vi "Simulated Car Client.vi"(7 "stop signal":refnum<user-event>, 10 "project namespace":string="LabVIEWDemo", 11 "Client Name":string="Car") -> ()   [LabVIEW 2017]
uses:
  Car/Car State -- enum.ctl
  <vilib>/LabVIEW Open Source Project/MQTT Broker/Client/Client.lvclass
  C:/Program Files (x86)/National Instruments/LabVIEW 2017/vi.lib/LabVIEW Open Source Project/MQTT Broker/MQTT_Base/MQTT_Base.lvclass
  <vilib>/LabVIEW Open Source Project/MQTT Broker/Control Packets/PUBLISH/PUBLISH.lvclass
  C:/Program Files (x86)/National Instruments/LabVIEW 2017/vi.lib/LabVIEW Open Source Project/MQTT Broker/Control Packets/ControlPacket/ControlPacket.lvclass
  Node Type -- enum.ctl
  TrafficMap/TrafficMap.lvclass
  RequestPayload -- cluster.ctl
  TrafficMap/TrafficMap.lvclass/TrafficMap.ctl
  ResponsePayload -- cluster.ctl
  Serializer.JKI-JSON/Serializer.JKI-JSON.lvclass
  C:/Program Files (x86)/National Instruments/LabVIEW 2017/vi.lib/LabVIEW Open Source Project/Serializer/Serializer/Serializer.lvclass
  <vilib>/LabVIEW Open Source Project/MQTT Broker/MQTT_Base/MQTT_Base.lvclass/MQTT_Base.ctl
  <vilib>/LabVIEW Open Source Project/MQTT Broker/Client/Client.lvclass/Client.ctl
  <vilib>/LabVIEW Open Source Project/MQTT Broker/Control Packets/CONNECT/ConnectFlags -- cluster.ctl
  ConnectPayload-- cluster.ctl
  DisconnectPayload-- cluster.ctl
  <vilib>/LabVIEW Open Source Project/MQTT Broker/Control Packets/ControlPacket/ControlPacket.lvclass/ControlPacket.ctl
  0d705227-134d-4031-8d1e-e35da49b8ba8.vi
  580889ff-0a4c-41a4-b259-1db762517910.vi
  3d3687d4-2784-4a3f-94ff-e25152285f29.vi
  45bbbbd6-bbd6-4c9d-8aa1-54a553140d59.vi
  a8e81dbf-d079-406f-abbd-3f6e0d275bc5.vi
  b830538a-2e83-4cc7-9605-dce1a29f0d38.vi
  <vilib>/LabVIEW Open Source Project/Serializer/Serializer.FlattenedString/Serializer.FlattenedString.lvclass
  <vilib>/LabVIEW Open Source Project/MQTT Broker/MQTT_Base/Decode Publish Package.vi
  <vilib>/LabVIEW Open Source Project/Serializer/Serializer/Serializer.lvclass
  <vilib>/LabVIEW Open Source Project/MQTT Broker/MQTT_Base/MQTT_Base.lvclass
  <vilib>/LabVIEW Open Source Project/MQTT Broker/Control Packets/ControlPacket/ControlPacket.lvclass
  <vilib>/LabVIEW Open Source Project/MQTT Broker/Control Packets/CONNECT/CONNECT.lvclass
  <vilib>/addons/_JKI.lib/Serialization/JSON/JKI JSON Serialization.lvlib
  Car/Car.lvclass
panel:
  in  "Map Update":bool
  out "Map":u16[][](graph)
  in  "Zones":u16(ring) items=["A", "B", "C", "D"]
  in  "Set Zone":bool
  in  "car state":T1
  in  "List Zones":bool
  out "Raw Packet String":string
  out "Payload":variant
  in  "Car Client Status":i32(listbox)
  out "Topic":string
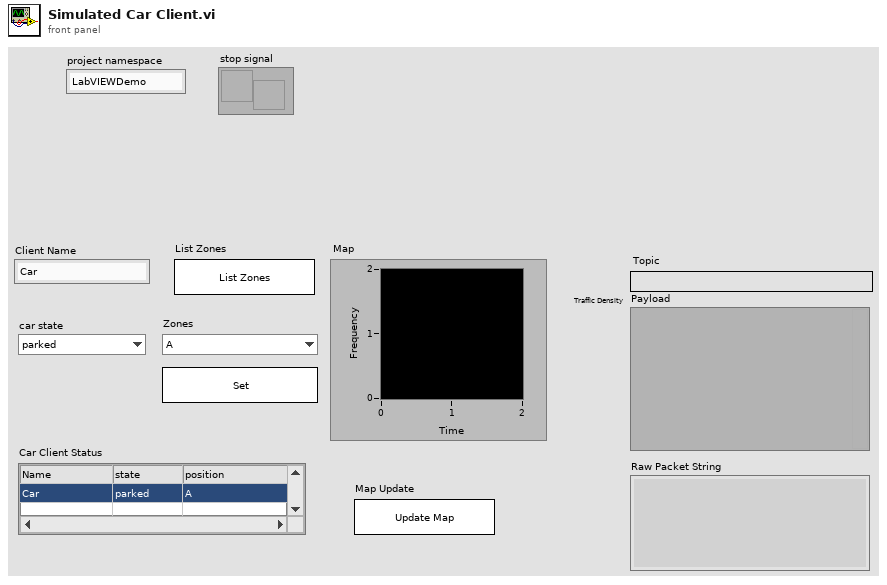
[diagram p1: front panel]
types:
  T1 = typedef "Car.lvclass/Car State -- enum.ctl" = enum16{"parked", "driving"}
  T2 = enum32{"Invalid", "Standard", "Closed", "Hidden", "Minimized", "Maximized"}
  T3 = enum32{"invalid app kind", "Development System", "Run Time System", "Student Edition", "Embedded LabVIEW", "Evaluation", "Custom"}
  T4 = typedef "ResponsePayload -- cluster.ctl" = cluster{"request":string, "reply":variant}
  T5 = typedef "CONNECT.lvclass/ConnectFlags -- cluster.ctl" = cluster{"Reserved":bool, "Clean Session":bool, "Will Flag":bool, "Will QoS 1":bool, "Will QoS 2":bool, "Will Retain":bool, "Password Flag":bool, "User Name Flag":bool}
  T6 = cluster{"Will Topic":string, "Will Message":string, "Username":string, "Password":string}
  T7 = typedef "RequestPayload -- cluster.ctl" = cluster{"request":string, "reply-to":string}
  T8 = typedef "ConnectPayload-- cluster.ctl" = cluster{"Node type":string}
  T9 = typedef "DisconnectPayload-- cluster.ctl" = cluster{"timestamp":string}
  T10 = typedef "Node Type -- enum.ctl" = enum16{"Car", "Hub", "Sensor", "Relay"}
  T11 = cluster{"Core":cluster{"Current VI Reference":refnum<vi>, "Close Panel on Exit?":bool}, "server address":string, "project namespace":string, "Client Name":string, "Node type":T10, "Client":refnum<class "Client.lvclass">, "Close on MQTT Disconnection?":bool, "Hub Name":string, "AppMessage":refnum<class "PUBLISH.lvclass">, "stop signal":refnum<user-event>, "TrafficMap":refnum<class "TrafficMap.lvclass">, "Request":T7}
  T12 = cluster{"Current VI Reference":refnum<vi>, "Close Panel on Exit?":bool}
  T13 = typedef "MQTT Server.lvlib/Client.lvclass/Public Events -- cluster.ctl" = cluster{"Connection Status":refnum<user-event>, "Connected":refnum<user-event>, "Application Message":refnum<user-event>}
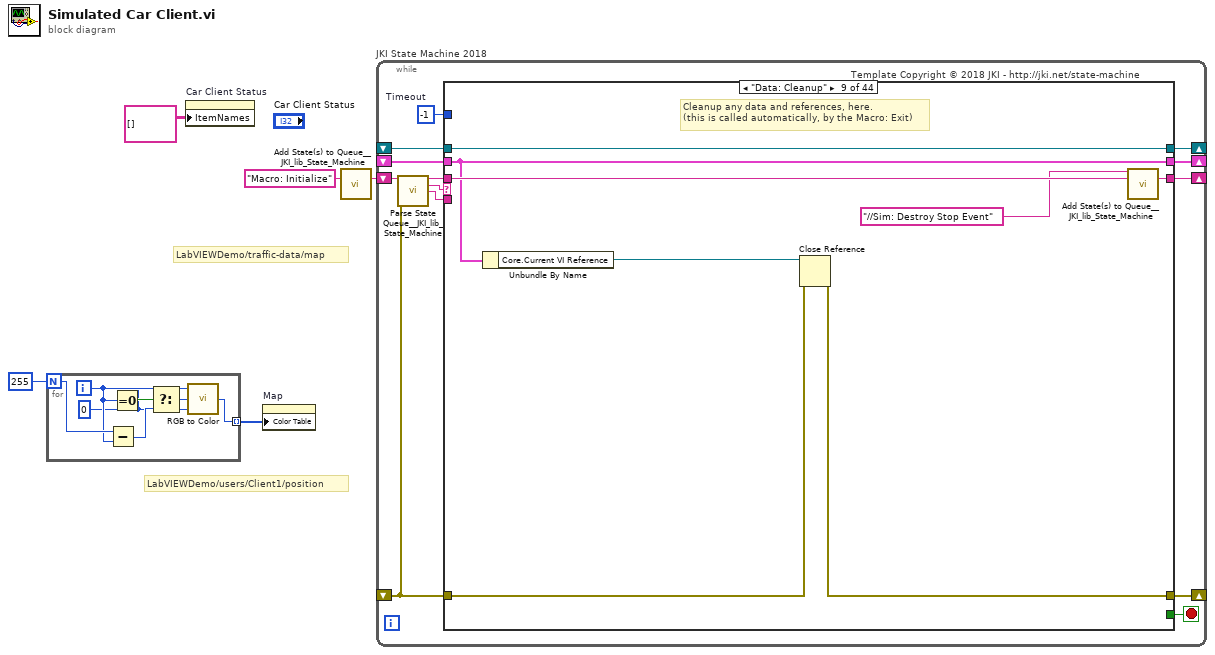
[diagram p0: block diagram]
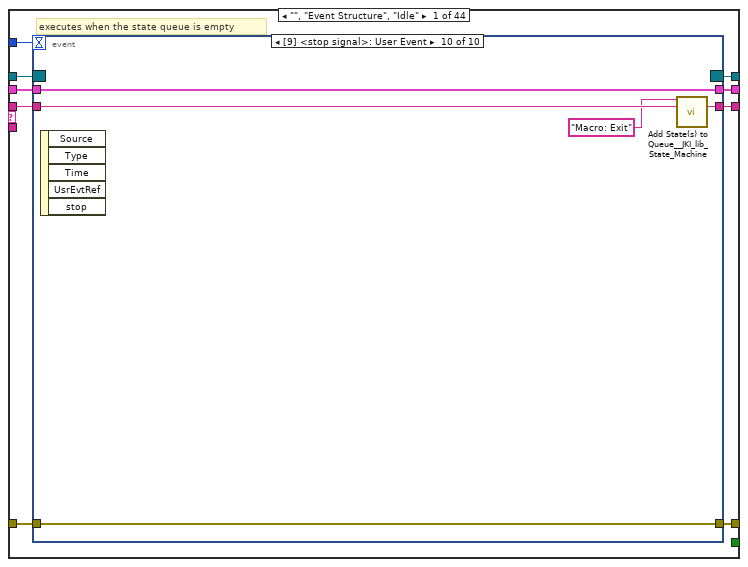
[diagram p2: hidden frame]
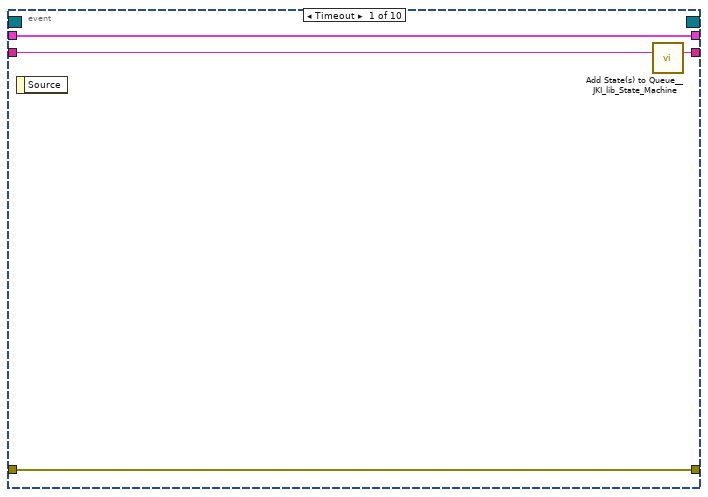
[diagram p3: hidden frame]
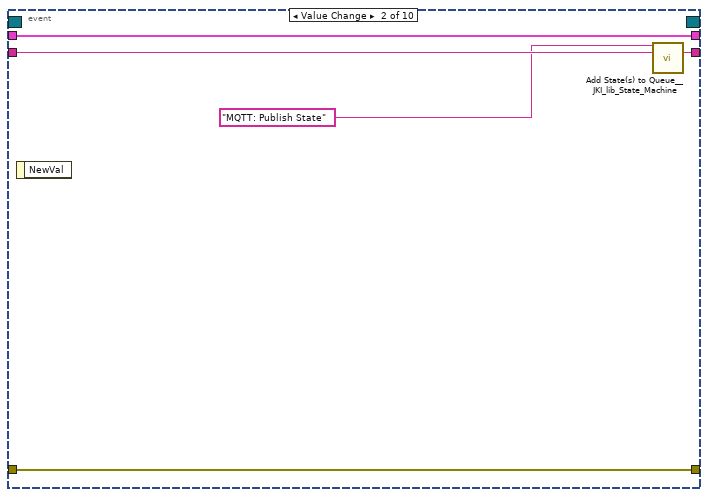
[diagram p4: hidden frame]
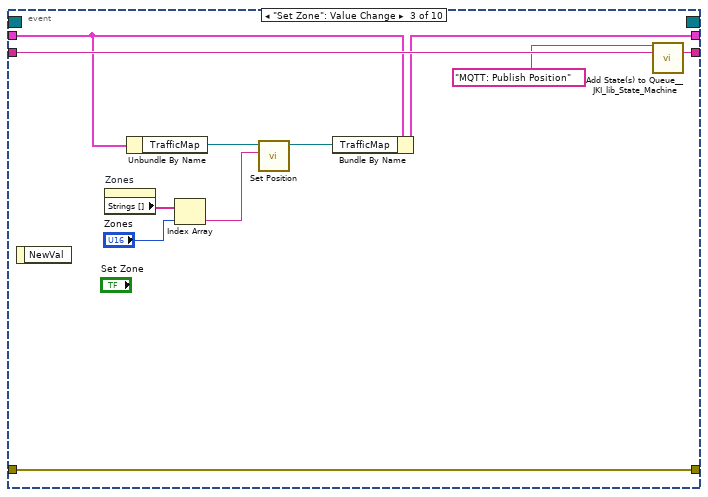
[diagram p5: hidden frame]
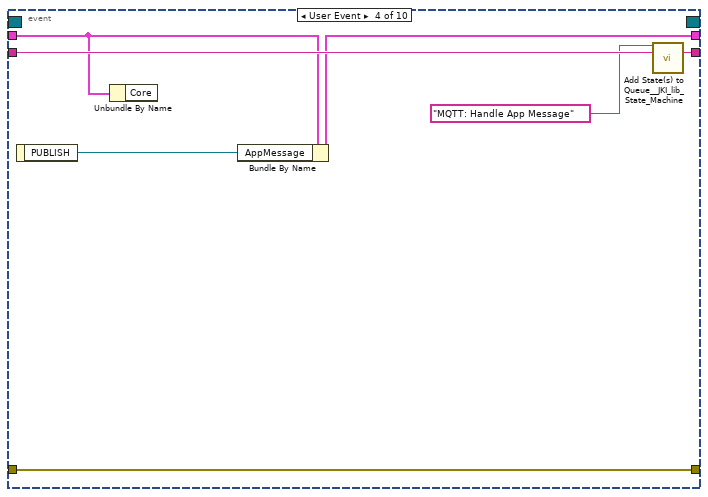
[diagram p6: hidden frame]
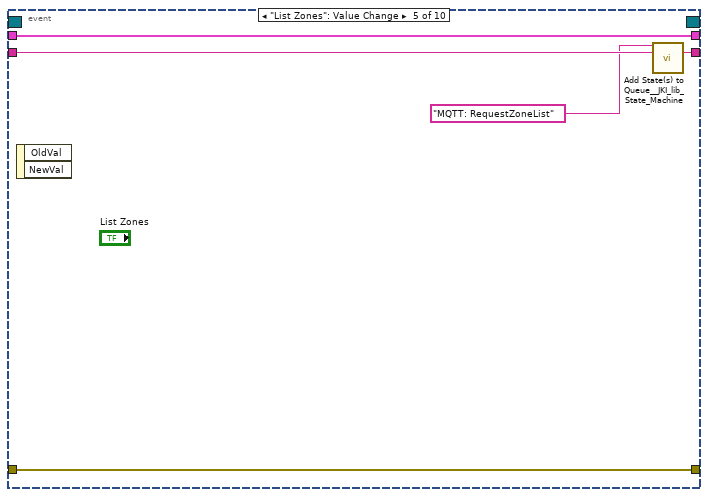
[diagram p7: hidden frame]
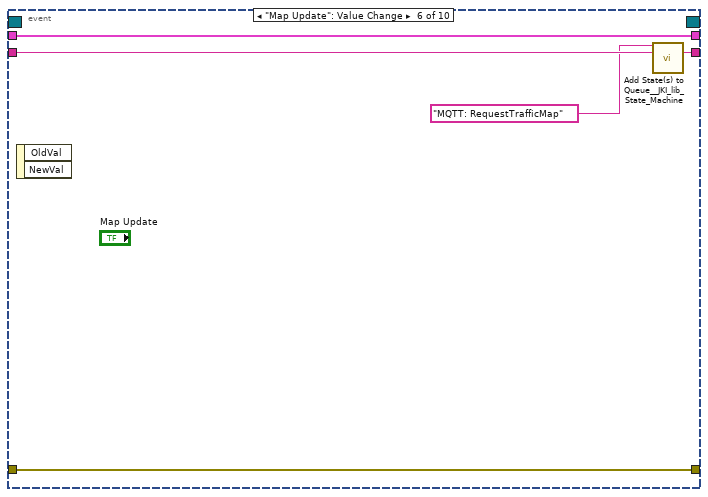
[diagram p8: hidden frame]
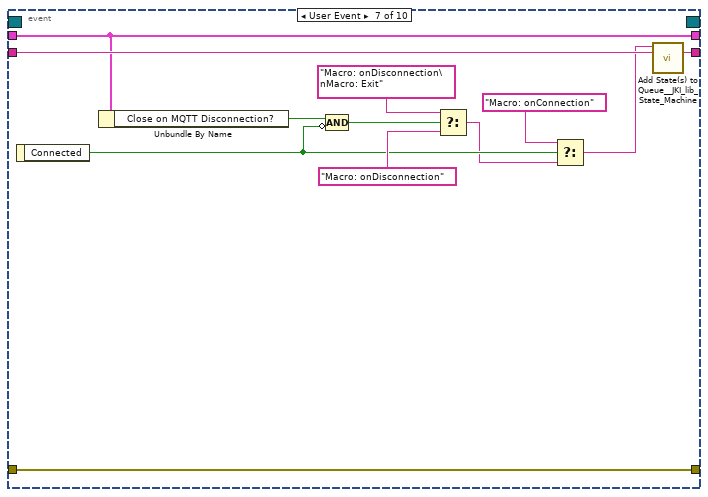
[diagram p9: hidden frame]
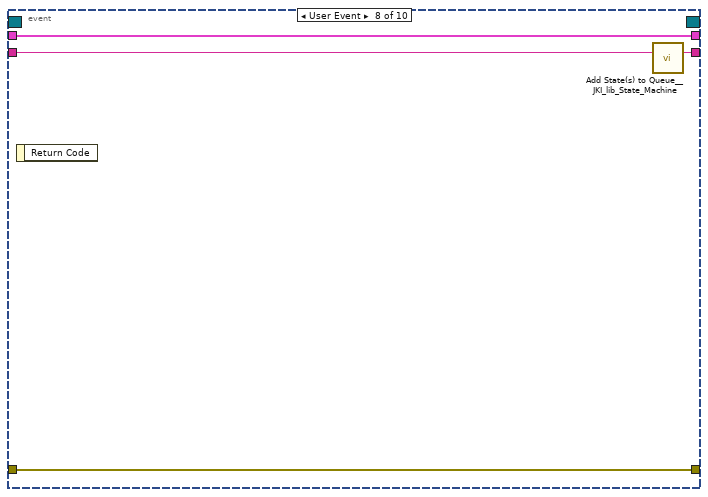
[diagram p10: hidden frame]
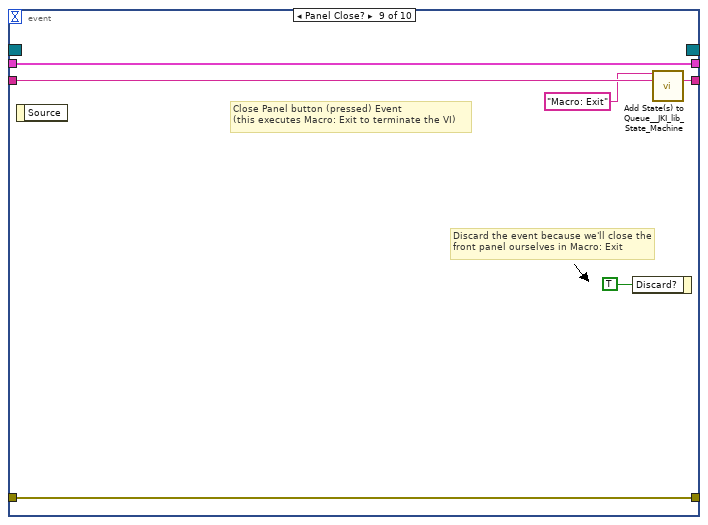
[diagram p11: hidden frame]
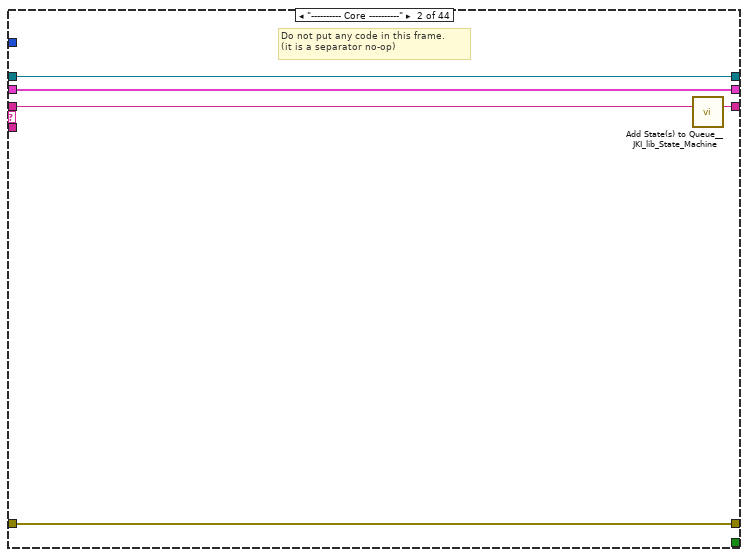
[diagram p12: hidden frame]
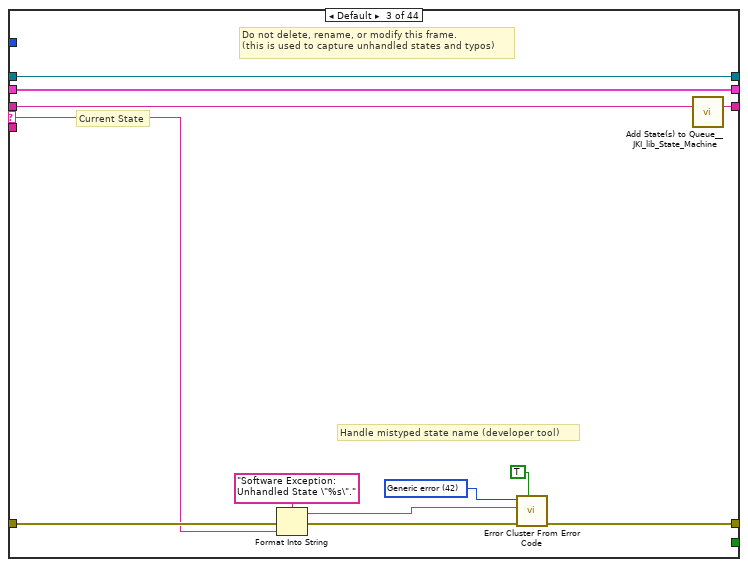
[diagram p13: hidden frame]
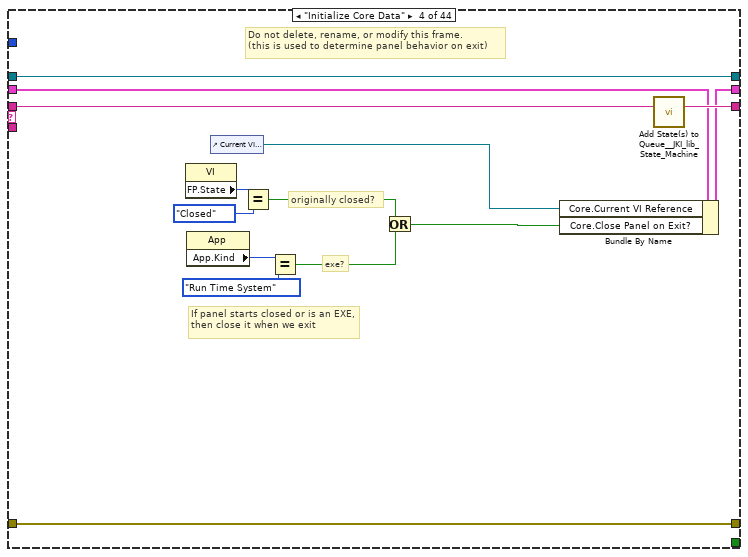
[diagram p14: hidden frame]
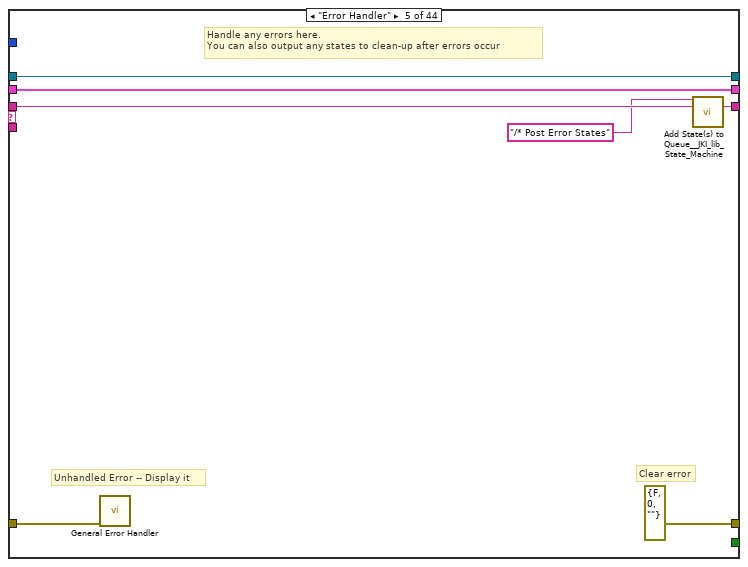
[diagram p15: hidden frame]
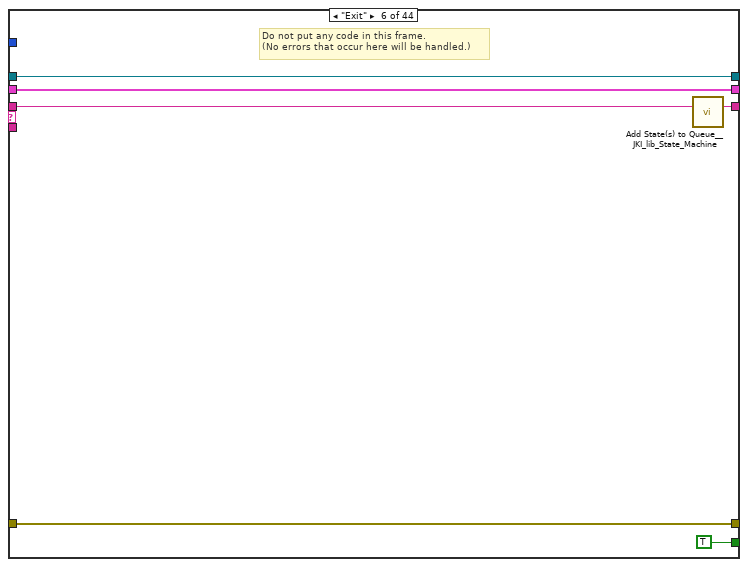
[diagram p16: hidden frame]
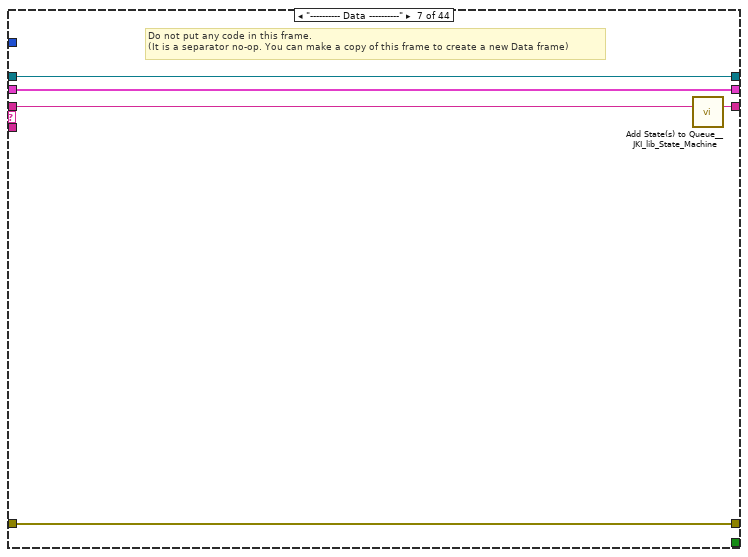
[diagram p17: hidden frame]
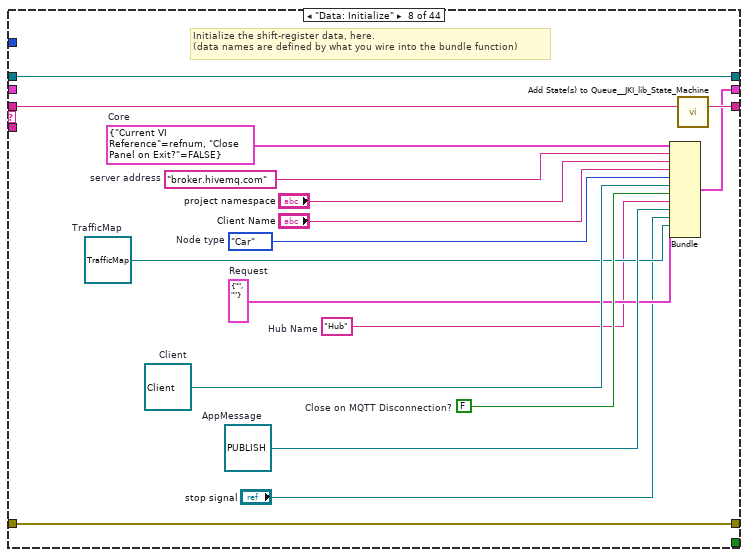
[diagram p18: hidden frame]
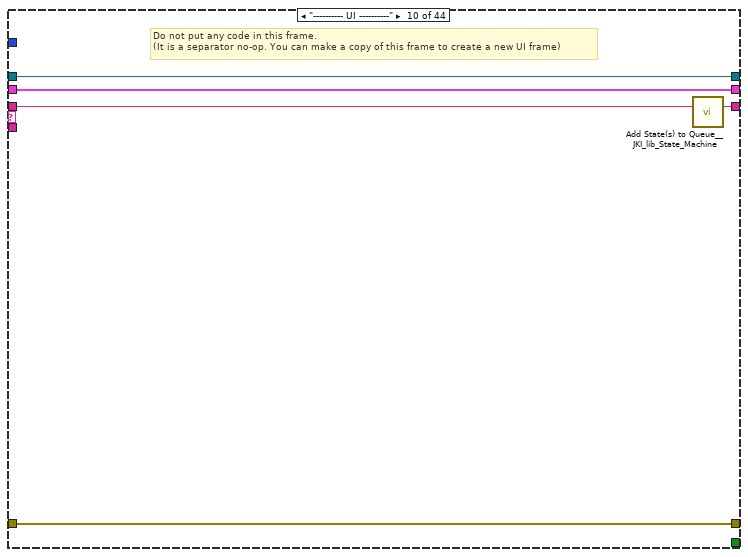
[diagram p19: hidden frame]
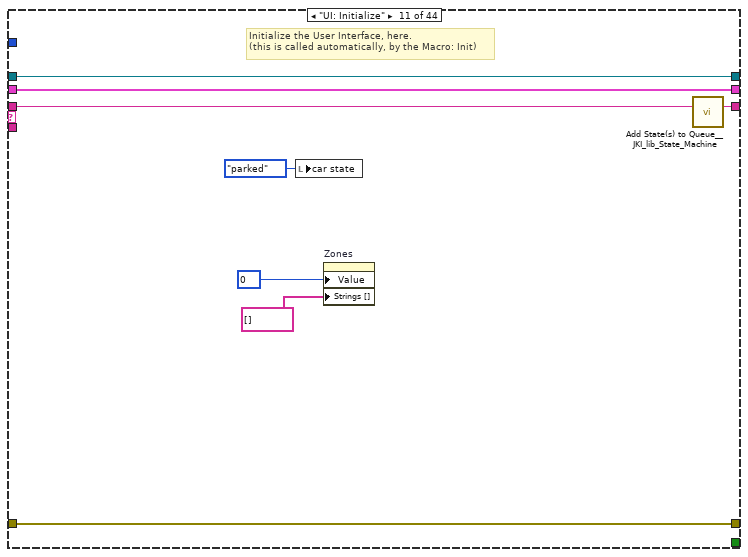
[diagram p20: hidden frame]
diagram:
  # "LabVIEWDemo/traffic-data/map"
  # "LabVIEWDemo/users/Client1/position"
  n1 = for {
    N: 255 -> [w11]
    tunnel: [w12] -> w1 mode=indexing
    i -> [w10]
    w7 = u8 0 ("B")
    n2 = Subtract(x=w11, y=w10) -> (x-y=w8:i32)
    n3 = Equal To 0?(x=w10) -> (x = 0?=w9:bool)
    n4 = Select(t=w7, s=w9, f=w8) -> (s? t:f=w6:i32)
    n5 = call <vilib>:"RGB to Color.vi"("B"=w7, "G"=w6, "R"=w10) -> ("Color"=w12:u32)
  }
  n6 = property on="Car Client Status" class="MCListbox (strict)"("ItemNames"=string[][] [] ("Item Names")) -> ()  [unwired: 2 in, 2 out]
  n7 = property on="Map" class="IntGraph (strict)"("Color Table"=w1) -> ()  [unwired: 2 in, 2 out]
  n8 = call <vilib>:"Add State(s) to Queue__JKI_lib_State_Machine.vi"("State(s) in (\"\")"="Macro: Initialize") -> ("States Out"=w4:string)  [unwired: 14 in]
  n9 = while "JKI State Machine 2018" {
    shift-right: [w18] -> _
    shift-left: _ -> [w17]
    shift-right: [w21] -> _
    shift-left: _ -> [w15]
    shift-right: [w20] -> _
    shift-left: w4 -> [w22]
    shift-right: [w14] -> _
    shift-left: _ -> [w13]
    stop <- w19 stop-if-true
    w16 = -1  # Timeout
    # "Template Copyright © 2018 JKI - http://jki.net/state-machine"
    n10 = call <vilib>:"Parse State Queue__JKI_lib_State_Machine.vi"("State Queue"=w22, "Error In (no error)"=w15) -> ("Remaining States"=w24:string, "Current State"=w25:string, "Arguments"=w23:string)  [unwired: 11 in]
    n11 = case shown="\"Data: Cleanup\"" w25 {
      selector: w25 -> [_ _ w105 _ _ _ _ _ _ _ _ _ _ _ _ _ _ _ _ _ _ _ _ _ _ _ _ _ _ _ _ _ _ _ _ _ _ _ _ _ _ _ _ _]
      tunnel: w24 -> [w34 w103 w109 w129 w136 w142 w147 w164 w172 w177 w185 w192 w199 w206 w218 w288 w294 w300 w306 w311 w317 w329 w334 w342 w348 w355 w360 w375 w396 w407 w419 w443 w456 w469 w484 w499 w517 w535 w552 w568 w589 w747 w753 w760]
      tunnel: w23 -> [_ _ _ _ _ _ _ _ _ _ _ _ _ w201 w212 _ _ _ _ _ _ _ _ _ _ _ _ _ _ _ _ _ _ _ _ _ _ _ _ _ _ _ _ _]
      tunnel: w17 -> [w32 w100 w107 w122 w133 w140 w144 _ w167 w174 w183 w188 w195 w204 w214 w285 w291 w297 w303 w308 w314 w326 w331 w336 w344 w351 w357 w362 w393 w405 w416 w440 w453 w466 w481 w496 w514 w532 w549 w565 w575 w744 w748 w758]
      tunnel: [w31 w101 w111 w126 errorcluster {"status"=FALSE, "code"=0, "source"=""} ("error out") w139 w145 w161 w168 w175 w182 w190 w197 w202 w215 w286 w292 w298 w304 w309 w315 w327 w332 w340 w346 w353 w358 w366 w394 w397 w409 w434 w445 w461 w472 w487 w507 w525 w540 w556 w586 w739 w749 w755] -> w21
      tunnel: w15 -> [w30 w101 w110 w126 w132 w139 w145 w161 w169 w175 w182 w190 w197 w203 w216 w286 w292 w298 w304 w309 w315 w327 w332 w340 w346 w353 w358 w367 w394 w403 w412 w435 w446 w462 w473 w488 w508 w526 w541 w557 w586 w737 w750 w756]
      tunnel: [w33 w102 w108 w128 w135 w141 w146 w163 w171 w176 w184 w191 w198 w205 w217 w287 w293 w299 w305 w310 w316 w328 w333 w341 w347 w354 w359 w374 w395 w406 w418 w442 w455 w468 w483 w498 w516 w534 w551 w567 w588 w746 w752 w759] -> w20
      tunnel: [_ _ _ _ _ TRUE _ _ _ _ _ _ _ _ _ _ _ _ _ _ _ _ _ _ _ _ _ _ _ _ _ _ _ _ _ _ _ _ _ _ _ _ _ _] -> w19
      tunnel: [w29 w100 w107 w127 w133 w140 w144 w162 w167 w174 w183 w188 w195 w204 w214 w285 w291 w297 w303 w308 w314 w326 w331 w335 w344 w351 w357 w373 w393 w404 w417 w441 w454 w467 w482 w497 w515 w533 w550 w566 w574 w745 w748 w758] -> w18
      tunnel: w16 -> [w28 _ _ _ _ _ _ _ _ _ _ _ _ _ _ _ _ _ _ _ _ _ _ _ _ _ _ _ _ _ _ _ _ _ _ _ _ _ _ _ _ _ _ _]
      tunnel: w13 -> [w27 w99 w104 w116 w130 w137 w143 w156 w166 w173 w181 w189 w196 w200 w211 w284 w289 w295 w301 w307 w312 w318 w330 w339 w345 w352 w356 w372 w392 w402 _ w439 w452 w465 w480 w495 w513 w531 w548 w564 w587 w743 w751 w754]
      tunnel: [w26 w99 w104 w116 w130 w137 w143 w156 w166 w173 w181 w189 w196 w200 w211 w284 w289 w295 w301 w307 w312 w318 w330 w339 w345 w352 w356 w372 w392 w402 w411 w439 w452 w465 w480 w495 w513 w531 w548 w564 w587 w743 w751 w754] -> w14
      frame "", "Event Structure", "Idle" {
        # "executes when the state queue is empty"
        n12 = event shown="[9] <stop signal>: User Event" {
          selector: w27 -> [_ _ _ _ _ _ _ _ _ _]
          dyn-events: [_ _ _ _ _ _ _ _ _ _] -> w26
          timeout: w28 -> [_ _ _ _ _ _ _ _ _ _]
          tunnel: w34 -> [w38 w43 w54 w61 w66 w71 w83 w87 w93 w98]
          tunnel: [w37 w42 w53 w60 w65 w70 w82 w86 w92 w97] -> w33
          tunnel: w32 -> [w35 w40 w50 w57 w62 w67 w80 w84 w90 w95]
          tunnel: [w36 w41 w52 w59 w64 w69 w81 w85 w91 w96] -> w31
          tunnel: w30 -> [w36 w41 w52 w59 w64 w69 w81 w85 w91 w96]
          tunnel: [w35 w40 w49 w56 w62 w67 w80 w84 w90 w95] -> w29
          event Timeout {
            n13 = event-data() -> ()  [unwired: 1 in, 1 out]
            n14 = call <vilib>:"Add State(s) to Queue__JKI_lib_State_Machine.vi"("State(s) in (\"\")"=w38) -> ("States Out"=w37:string)  [unwired: 14 in]
          }
          event Value Change {
            n15 = event-data() -> ()  [unwired: 1 in, 1 out]
            n16 = call <vilib>:"Add State(s) to Queue__JKI_lib_State_Machine.vi"("State(s) in Front (\"\")"="MQTT: Publish State", "State(s) in (\"\")"=w43) -> ("States Out"=w42:string)  [unwired: 13 in]
          }
          event "Set Zone": Value Change {
            n17 = event-data() -> ()  [unwired: 1 in, 1 out]
            n18 = property on="Zones" class="Ring (strict)"() -> ("Strings []"=w46:string[])  [unwired: 2 in, 2 out]
            n19 = Unbundle By Name(w50) -> ("TrafficMap"=w48:refnum<class "TrafficMap.lvclass">)
            n20 = Index Array(array=w46, index="Zones") -> (element=w44:string)
            n21 = call "Set Position.vi"("Position"=w44, "TrafficMap in"=w48) -> ("TrafficMap out"=w47:refnum<class "TrafficMap.lvclass">)  [unwired: 8 in, 1 out]
            n22 = Bundle By Name(cluster=w50, "TrafficMap"=w47) -> (w49:T11)
            n23 = call <vilib>:"Add State(s) to Queue__JKI_lib_State_Machine.vi"("State(s) in Front (\"\")"="MQTT: Publish Position", "State(s) in (\"\")"=w54) -> ("States Out"=w53:string)  [unwired: 13 in]
          }
          event User Event {
            n24 = event-data() -> ("PUBLISH"=w58:refnum<class "PUBLISH.lvclass">)  [unwired: 1 in]
            n25 = Unbundle By Name(w57) -> ()  [unwired: 1 out]
            n26 = Bundle By Name(cluster=w57, "AppMessage"=w58) -> (w56:T11)
            n27 = call <vilib>:"Add State(s) to Queue__JKI_lib_State_Machine.vi"("State(s) in Front (\"\")"="MQTT: Handle App Message", "State(s) in (\"\")"=w61) -> ("States Out"=w60:string)  [unwired: 13 in]
          }
          event "List Zones": Value Change {
            n28 = event-data() -> ()  [unwired: 1 in, 2 out]
            n29 = call <vilib>:"Add State(s) to Queue__JKI_lib_State_Machine.vi"("State(s) in Front (\"\")"="MQTT: RequestZoneList", "State(s) in (\"\")"=w66) -> ("States Out"=w65:string)  [unwired: 13 in]
          }
          event "Map Update": Value Change {
            n30 = event-data() -> ()  [unwired: 1 in, 2 out]
            n31 = call <vilib>:"Add State(s) to Queue__JKI_lib_State_Machine.vi"("State(s) in Front (\"\")"="MQTT: RequestTrafficMap", "State(s) in (\"\")"=w71) -> ("States Out"=w70:string)  [unwired: 13 in]
          }
          event User Event {
            n32 = event-data() -> ("Connected"=w75:bool)  [unwired: 1 in]
            n33 = Unbundle By Name(w80) -> ("Close on MQTT Disconnection?"=w79:bool)
            n34 = Compound Arithmetic op=AND(w79, invert w75) -> (w78:bool)
            n35 = Select(t="Macro: onDisconnection\nMacro: Exit", s=w78, f="Macro: onDisconnection" ("t")) -> (s? t:f=w73:string)
            n36 = Select(t="Macro: onConnection", s=w75, f=w73) -> (s? t:f=w72:string)
            n37 = call <vilib>:"Add State(s) to Queue__JKI_lib_State_Machine.vi"("State(s) in Front (\"\")"=w72, "State(s) in (\"\")"=w83) -> ("States Out"=w82:string)  [unwired: 13 in]
          }
          event User Event {
            n38 = event-data() -> ()  [unwired: 1 in, 1 out]
            n39 = call <vilib>:"Add State(s) to Queue__JKI_lib_State_Machine.vi"("State(s) in (\"\")"=w87) -> ("States Out"=w86:string)  [unwired: 14 in]
          }
          event Panel Close? {
            # "Discard the event because we'll close the front panel ourselves in Macro: Exit"
            # "Close Panel button (pressed) Event\n(this executes Macro: Exit to terminate the VI)"
            n40 = event-data() -> ()  [unwired: 1 in, 1 out]
            n41 = event-data("Discard?"=TRUE) -> ()  [unwired: 1 in, 1 out]
            n42 = call <vilib>:"Add State(s) to Queue__JKI_lib_State_Machine.vi"("State(s) in Front (\"\")"="Macro: Exit", "State(s) in (\"\")"=w93) -> ("States Out"=w92:string)  [unwired: 13 in]
          }
          event User Event {
            n43 = event-data() -> ()  [unwired: 1 in, 5 out]
            n44 = call <vilib>:"Add State(s) to Queue__JKI_lib_State_Machine.vi"("State(s) in Front (\"\")"="Macro: Exit", "State(s) in (\"\")"=w98) -> ("States Out"=w97:string)  [unwired: 13 in]
          }
        }
      }
      frame "---------- Core ----------" {
        # "Do not put any code in this frame.\n(it is a separator no-op)"
        n45 = call <vilib>:"Add State(s) to Queue__JKI_lib_State_Machine.vi"("State(s) in (\"\")"=w103) -> ("States Out"=w102:string)  [unwired: 14 in]
      }
      frame Default {
        w114 = 42 items=["No error", "Argument error", "Memory is full", "Out of zone", "End of file", "File already open", "Generic file I/O error", "File not found", "File permission error", "Disk is full", "Duplicate path", "Too many files open", "System feature not enabled", "Resource file not found", "Cannot add resource", "Resource not found", "Image not found", "Image memory error", "Pen does not exist", "Config type invalid", "Config token not found", "Config parse error", "Config memory error", "Bad external code format", "Bad external code offset", "External code not present", "Null window", "Destroy window error", "Null menu", "Print aborted", "Bad print record", "Print driver error", "Windows error during printing", "Memory error during printing", "Print dialog error", "Generic print error", "Invalid device refnum", "Device not found", "Device parameter error", "Device unit error", "Cannot open device", "Device call aborted", "Generic error", "Cancelled by user", "Object ID too low", "Object ID too high", "Object not in heap", "Unknown heap", "Unknown object (invalid DefProc)", "Unknown object (DefProc not in table)", "Message out of range", "Invalid (null) method", "Unknown message", "Manager call not supported", "Bad address", "Network operation in progress", "Network operation timed out", "Connection is busy", "Network attribute not supported", "Network error", "Address in use", "System out of memory", "Connection aborted", "Connection refused", "Not connected", "Already connected", "Connection closed", "Initialization error (interapplication manager)", "Bad occurrence", "Wait on unbound occurrence handler", "Occurrence queue overflow", "Datalog type conflict", "Unused", "Unrecognized type (interapplication manager)", "Memory corrupt", "Failed to make temporary DLL", "Old CIN version", "Drag socket not found", "Failed to load drop-object", "Failed to register OLE object", "Failed to release OLE object", "Format specifier type mismatch", "Unknown format specifier", "Too few format specifiers", "Too many format specifiers", "Scan failed", "Newer CIN version", "Error converting to variant", "Runtime menu error", "Password tampered", "Variant attribute not found", "Incompatible variant data type", "Event data is not available", "Event Store is not present", "Occurrence is not found", "Event Queue is not created", "Event info is not available", "Refnum passed is NULL", "Error retrieving Class GUID", "Error retrieving CoClass GUID", "Error retrieving TypeLib GUID.", "Bad built application magic bytes.", "Specific driver is different from the specific driver associated with the Logical Name.", "There is no session opened to the class driver.", "Max Error", "MAX - Error with config objects", "MAX - Error loading configuration", "MAX - Group not supported"]
        # "Current State"
        # "Do not delete, rename, or modify this frame.\n(this is used to capture unhandled states and typos)"
        # "Handle mistyped state name (developer tool)"
        n46 = Format Into String(format string="Software Exception: Unhandled State \"%s\"." ("message"), error in=w110, w105) -> (resulting string=w113:string, error out=w112:errorcluster)  [unwired: 1 in]
        n47 = call <vilib>:"Error Cluster From Error Code.vi"("show call chain? (False)"=TRUE, "error in (no error)"=w112, "error message (\"\")"=w113, "error code (0)"=w114) -> ("error out"=w111:errorcluster)  [unwired: 5 in]
        n48 = call <vilib>:"Add State(s) to Queue__JKI_lib_State_Machine.vi"("State(s) in (\"\")"=w109) -> ("States Out"=w108:string)  [unwired: 14 in]
      }
      frame "Initialize Core Data" {
        # "Do not delete, rename, or modify this frame.\n(this is used to determine panel behavior on exit)"
        # "originally closed?"
        # "exe?"
        # "If panel starts closed or is an EXE, then close it when we exit"
        n49 = property class="VI"() -> ("FP.State"=w119:T2)  [unwired: 2 in, 2 out]
        n50 = property class="App"() -> ("App.Kind"=w125:T3)  [unwired: 2 in, 2 out]
        n51 = control-ref of="Current VI Reference"() -> (w120:refnum<vi>)
        n52 = Equal?(x=w119, y=T2."Closed" ("Front Panel Window:State")) -> (x = y?=w117:bool)
        n53 = Equal?(x=w125, y=T3."Run Time System" ("Application:Kind")) -> (x = y?=w123:bool)
        n54 = Or(x=w117, y=w123) -> (x .or. y?=w121:bool)
        n55 = Bundle By Name(cluster=w122, "Core.Current VI Reference"=w120, "Core.Close Panel on Exit?"=w121) -> (w127:T11)
        n56 = call <vilib>:"Add State(s) to Queue__JKI_lib_State_Machine.vi"("State(s) in (\"\")"=w129) -> ("States Out"=w128:string)  [unwired: 14 in]
      }
      frame "Error Handler" {
        # "Unhandled Error -- Display it"
        # "Handle any errors here.\nYou can also output any states to clean-up after errors occur"
        # "Clear error"
        n57 = call <vilib>:"General Error Handler.vi"("error in (no error)"=w132) -> ()  [unwired: 10 in, 5 out]
        n58 = call <vilib>:"Add State(s) to Queue__JKI_lib_State_Machine.vi"("State(s) in Front (\"\")"="/* Post Error States", "State(s) in (\"\")"=w136) -> ("States Out"=w135:string)  [unwired: 13 in]
      }
      frame "Exit" {
        # "Do not put any code in this frame.\n(No errors that occur here will be handled.)"
        n59 = call <vilib>:"Add State(s) to Queue__JKI_lib_State_Machine.vi"("State(s) in (\"\")"=w142) -> ("States Out"=w141:string)  [unwired: 14 in]
      }
      frame "---------- Data ----------" {
        # "Do not put any code in this frame.\n(It is a separator no-op. You can make a copy of this frame to create a new Data frame)"
        n60 = call <vilib>:"Add State(s) to Queue__JKI_lib_State_Machine.vi"("State(s) in (\"\")"=w147) -> ("States Out"=w146:string)  [unwired: 14 in]
      }
      frame "Data: Initialize" {
        w150 = "Hub"  # Hub Name
        w151 = T7 {"request"="", "reply-to"=""}  # Request
        w152 = refnum<class "TrafficMap.lvclass"> refnum  # TrafficMap
        w153 = Node_Type_--_enum."Car"  # Node type
        w154 = refnum<class "PUBLISH.lvclass"> refnum  # AppMessage
        w155 = FALSE  # Close on MQTT Disconnection?
        w157 = refnum<class "Client.lvclass"> refnum  # Client
        w158 = "broker.hivemq.com"  # server address
        w159 = T12 {"Current VI Reference"=refnum, "Close Panel on Exit?"=FALSE}  # Core
        # "Initialize the shift-register data, here.\n(data names are defined by what you wire into the bundle function)"
        n61 = Bundle("Core"=w159, "server address"=w158, "project namespace"="project namespace", "Client Name"="Client Name", "Node type"=w153, "Client"=w157, "Close on MQTT Disconnection?"=w155, "Hub Name"=w150, "AppMessage"=w154, "stop signal"="stop signal", "TrafficMap"=w152, "Request"=w151) -> (w162:T11)  [unwired: 1 in]
        n62 = call <vilib>:"Add State(s) to Queue__JKI_lib_State_Machine.vi"("State(s) in (\"\")"=w164) -> ("States Out"=w163:string)  [unwired: 14 in]
      }
      frame "Data: Cleanup" {
        # "Cleanup any data and references, here.\n(this is called automatically, by the Macro: Exit)"
        n63 = Unbundle By Name(w167) -> ("Core.Current VI Reference"=w170:refnum<vi>)
        n64 = Close Reference(reference=w170, error in (no error)=w169) -> (error out=w168:errorcluster)
        n65 = call <vilib>:"Add State(s) to Queue__JKI_lib_State_Machine.vi"("State(s) in Front (\"\")"="//Sim: Destroy Stop Event", "State(s) in (\"\")"=w172) -> ("States Out"=w171:string)  [unwired: 13 in]
      }
      frame "---------- UI ----------" {
        # "Do not put any code in this frame.\n(It is a separator no-op. You can make a copy of this frame to create a new UI frame)"
        n66 = call <vilib>:"Add State(s) to Queue__JKI_lib_State_Machine.vi"("State(s) in (\"\")"=w177) -> ("States Out"=w176:string)  [unwired: 14 in]
      }
      frame "UI: Initialize" {
        w179 = u16 0 items=[""] ("Zones")
        # "Initialize the User Interface, here.\n(this is called automatically, by the Macro: Init)"
        n67 = local write "car state"(Car_State_--_enum."parked" ("car state")) -> ()
        n68 = property on="Zones" class="Ring (strict)"("Value"=w179, "Strings []"=string[] [] ("Zones")) -> ()  [unwired: 2 in, 2 out]
        n69 = call <vilib>:"Add State(s) to Queue__JKI_lib_State_Machine.vi"("State(s) in (\"\")"=w185) -> ("States Out"=w184:string)  [unwired: 14 in]
      }
      frame "UI: Update Zone List" {
        n70 = Unbundle By Name(w188) -> ("TrafficMap"=w187:refnum<class "TrafficMap.lvclass">)
        n71 = call "List Zones.vi"("TrafficMap in"=w187) -> ("Zones"=w186:string[])  [unwired: 7 in, 3 out]
        n72 = property on="Zones" class="Ring (strict)"("Strings []"=w186) -> ()  [unwired: 2 in, 2 out]
        n73 = call <vilib>:"Add State(s) to Queue__JKI_lib_State_Machine.vi"("State(s) in (\"\")"=w192) -> ("States Out"=w191:string)  [unwired: 14 in]
      }
      frame "UI: Update Zone Map" {
        n74 = Unbundle By Name(w195) -> ("TrafficMap"=w194:refnum<class "TrafficMap.lvclass">)
        n75 = call "Read Map.vi"("TrafficMap in"=w194) -> ("Map"=→"Map":u16[][])  [unwired: 8 in, 2 out]
        n76 = call <vilib>:"Add State(s) to Queue__JKI_lib_State_Machine.vi"("State(s) in (\"\")"=w199) -> ("States Out"=w198:string)  [unwired: 14 in]
      }
      frame "UI: Cursor Set" {
        # "Argument"
        # "Set and Unset Cursor Busy.\n(Usage: \"UI: Cursor Set >> Busy|Idle\")"
        n77 = case shown="\"Idle\", Default" w201 {
          tunnel: w203 -> [w208 w210]
          tunnel: [w207 w209] -> w202
          frame "Idle", Default {
            n78 = call <vilib>:"Unset Busy.vi"("error in (no error)"=w208) -> ("error out"=w207:errorcluster)  [unwired: 10 in]
          }
          frame "Busy" {
            n79 = call <vilib>:"Set Busy.vi"("error in (no error)"=w210) -> ("error out"=w209:errorcluster)  [unwired: 9 in, 1 out]
          }
        }
        n80 = call <vilib>:"Add State(s) to Queue__JKI_lib_State_Machine.vi"("State(s) in (\"\")"=w206) -> ("States Out"=w205:string)  [unwired: 14 in]
      }
      frame "UI: Front Panel State" {
        # "Argument"
        # "Set Front Panel Open or Closed\n(Usage: \"UI: Front Panel State >> Open|Close\")"
        n81 = Unbundle By Name(w214) -> ("Core.Current VI Reference"=w213:refnum<vi>)
        n82 = case shown="\"Minimize\", \"Minimized\"" w212 {
          tunnel: w216 -> [w224 w239 w250 w263 w276]
          tunnel: [w226 w240 w252 w265 w278] -> w215
          tunnel: w213 -> [w225 w237 w251 w264 w277]
          frame "Open", "Standard", Default {
            w219 = T2."Standard" ("State")
            n83 = property class="VI"(reference=w225, error in=w224) -> (reference out=w222:refnum<vi>, error out=w223:errorcluster, "FP.State"=w221:T2)
            n84 = Not Equal?(x=w221, y=w219) -> (x != y?=w220:bool)
            n85 = case shown="True" w220 {
              tunnel: [w230 w232] -> w226
              tunnel: w223 -> [w229 w232]
              tunnel: w222 -> [w228 _]
              tunnel: w219 -> [w227 _]
              frame True {
                n86 = invoke class="VI" method="FP.Open"(reference=w228, error in=w229, "Activate"=TRUE, "State"=w227) -> (error out=w230:errorcluster)  [unwired: 1 in, 4 out]
              }
              frame False {
              }
            }
          }
          frame "Close", "Closed" {
            n87 = property class="VI"(reference=w237, error in=w239) -> (reference out=w236:refnum<vi>, error out=w238:errorcluster, "FP.State"=w234:T2)
            n88 = Not Equal?(x=w234, y=T2."Closed" ("Front Panel Window:State")) -> (x != y?=w233:bool)
            n89 = case shown="True" w233 {
              tunnel: [w241 w244] -> w240
              tunnel: w238 -> [w241 w243]
              tunnel: w236 -> [_ w242]
              frame False {
              }
              frame True {
                n90 = invoke class="VI" method="FP.Close"(reference=w242, error in=w243) -> (error out=w244:errorcluster)  [unwired: 1 in, 2 out]
              }
            }
          }
          frame "Hidden", "Hide" {
            w245 = T2."Hidden" ("State")
            n91 = property class="VI"(reference=w251, error in=w250) -> (reference out=w248:refnum<vi>, error out=w249:errorcluster, "FP.State"=w247:T2)
            n92 = Not Equal?(x=w247, y=w245) -> (x != y?=w246:bool)
            n93 = case shown="True" w246 {
              tunnel: [w256 w257] -> w252
              tunnel: w249 -> [w255 w257]
              tunnel: w248 -> [w254 _]
              tunnel: w245 -> [w253 _]
              frame True {
                n94 = invoke class="VI" method="FP.Open"(reference=w254, error in=w255, "State"=w253) -> (error out=w256:errorcluster)  [unwired: 2 in, 4 out]
              }
              frame False {
              }
            }
          }
          frame "Minimize", "Minimized" {
            w258 = T2."Minimized" ("State")
            n95 = property class="VI"(reference=w264, error in=w263) -> (reference out=w261:refnum<vi>, error out=w262:errorcluster, "FP.State"=w260:T2)
            n96 = Not Equal?(x=w260, y=w258) -> (x != y?=w259:bool)
            n97 = case shown="True" w259 {
              tunnel: [w269 w270] -> w265
              tunnel: w262 -> [w268 w270]
              tunnel: w261 -> [w267 _]
              tunnel: w258 -> [w266 _]
              frame True {
                n98 = invoke class="VI" method="FP.Open"(reference=w267, error in=w268, "State"=w266) -> (error out=w269:errorcluster)  [unwired: 2 in, 4 out]
              }
              frame False {
              }
            }
          }
          frame "Maximize", "Maximized" {
            w271 = T2."Maximized" ("State")
            n99 = property class="VI"(reference=w277, error in=w276) -> (reference out=w274:refnum<vi>, error out=w275:errorcluster, "FP.State"=w273:T2)
            n100 = Not Equal?(x=w273, y=w271) -> (x != y?=w272:bool)
            n101 = case shown="True" w272 {
              tunnel: [w282 w283] -> w278
              tunnel: w275 -> [w281 w283]
              tunnel: w274 -> [w280 _]
              tunnel: w271 -> [w279 _]
              frame True {
                n102 = invoke class="VI" method="FP.Open"(reference=w280, error in=w281, "State"=w279) -> (error out=w282:errorcluster)  [unwired: 2 in, 4 out]
              }
              frame False {
              }
            }
          }
        }
        n103 = call <vilib>:"Add State(s) to Queue__JKI_lib_State_Machine.vi"("State(s) in (\"\")"=w218) -> ("States Out"=w217:string)  [unwired: 14 in]
      }
      frame "---------- Macro ----------" {
        # "Do not put any code in this frame.\n(It is a separator no-op. You can make a copy of this frame to create a new Macro frame)"
        n104 = call <vilib>:"Add State(s) to Queue__JKI_lib_State_Machine.vi"("State(s) in (\"\")"=w288) -> ("States Out"=w287:string)  [unwired: 14 in]
      }
      frame "Macro: Initialize" {
        w290 = "Data: Initialize\nInitialize Core Data\n\nUI: Initialize\n//UI: Front Panel State >> Open\n//Sim: Create Stop Event\nMacro: MQTTConnect"  # Data: Initialize Initialize Core Data  UI: Initialize //UI: Front Panel State >> Open //Sim: Create Stop Event Macro: MQTTConnect
        # "Initialization Macro\n(This is called once, when the VI starts)"
        n105 = call <vilib>:"Add State(s) to Queue__JKI_lib_State_Machine.vi"("State(s) in Front (\"\")"=w290, "State(s) in (\"\")"=w294) -> ("States Out"=w293:string)  [unwired: 13 in]
      }
      frame "Macro: MQTTConnect" {
        n106 = call <vilib>:"Add State(s) to Queue__JKI_lib_State_Machine.vi"("State(s) in Front (\"\")"="MQTT: Create Client\nMQTT: Register for Events\nMQTT: Connect", "State(s) in (\"\")"=w300) -> ("States Out"=w299:string)  [unwired: 13 in]
      }
      frame "Macro: onConnection" {
        n107 = call <vilib>:"Add State(s) to Queue__JKI_lib_State_Machine.vi"("State(s) in Front (\"\")"="MQTT: Subscribe\nMQTT: PublishConnectionMessage\nMQTT: Publish State", "State(s) in (\"\")"=w306) -> ("States Out"=w305:string)  [unwired: 13 in]
      }
      frame "Macro: onDisconnection" {
        n108 = call <vilib>:"Add State(s) to Queue__JKI_lib_State_Machine.vi"("State(s) in (\"\")"=w311) -> ("States Out"=w310:string)  [unwired: 14 in]
      }
      frame "Macro: MQTTDisconnect" {
        n109 = call <vilib>:"Add State(s) to Queue__JKI_lib_State_Machine.vi"("State(s) in Front (\"\")"="MQTT: Unsubscribe\nMQTT: Unregister\nMQTT: PublishDisconnectionMessage\nMQTT: Disconnect\nMQTT: Destroy Client", "State(s) in (\"\")"=w317) -> ("States Out"=w316:string)  [unwired: 13 in]
      }
      frame "Macro: Exit" {
        # "Exit Macro\n(This is called once, when the VI exits)"
        n110 = Unbundle By Name(w326) -> ("Core.Close Panel on Exit?"=w325:bool)
        n111 = Select(t="UI: Front Panel State >> Close", s=w325, f="") -> (s? t:f=w322:string)
        n112 = call <vilib>:"Add State(s) to Queue__JKI_lib_State_Machine.vi"("State(s) in Front (\"\")"="//Sim: Send Stop Signal\nMacro: MQTTDisconnect", "State(s) in (\"\")"=w322, "State(s) at Back (\"\")"="Data: Cleanup\nExit") -> ("States Out"=w320:string)  [unwired: 12 in]
        n113 = call <vilib>:"Add State(s) to Queue__JKI_lib_State_Machine.vi"("State(s) in Front (\"\")"=w320, "State(s) in (\"\")"=w329) -> ("States Out"=w328:string)  [unwired: 13 in]
      }
      frame "---------- Simulation ----------" {
        # "Simulation Separator\n(You can make a copy of, or modify, this frame)"
        n114 = call <vilib>:"Add State(s) to Queue__JKI_lib_State_Machine.vi"("State(s) in (\"\")"=w334) -> ("States Out"=w333:string)  [unwired: 14 in]
      }
      frame "Sim: Create Stop Event" {
        w338 = FALSE  # stop
        n115 = Create User Event(user event datatype=w338) -> (user event=w337:refnum<user-event>)  [unwired: 1 in, 1 out]
        n116 = Bundle By Name(cluster=w336, "stop signal"=w337) -> (w335:T11)
        n117 = call <vilib>:"Add State(s) to Queue__JKI_lib_State_Machine.vi"("State(s) in (\"\")"=w342) -> ("States Out"=w341:string)  [unwired: 14 in]
      }
      frame "Sim: Destroy Stop Event" {
        n118 = Unbundle By Name(w344) -> ("stop signal"=w343:refnum<user-event>)
        n119 = Destroy User Event(user event=w343) -> ()  [unwired: 1 in, 1 out]
        n120 = call <vilib>:"Add State(s) to Queue__JKI_lib_State_Machine.vi"("State(s) in (\"\")"=w348) -> ("States Out"=w347:string)  [unwired: 14 in]
      }
      frame "Sim: Send Stop Signal" {
        n121 = Unbundle By Name(w351) -> ("stop signal"=w350:refnum<user-event>)
        n122 = Generate User Event(user event=w350, event data cluster=TRUE ("event data")) -> ()  [unwired: 2 in, 2 out]
        n123 = call <vilib>:"Add State(s) to Queue__JKI_lib_State_Machine.vi"("State(s) in (\"\")"=w355) -> ("States Out"=w354:string)  [unwired: 14 in]
      }
      frame "---------- Requests ----------" {
        # "Handling Requests\n(You can make a copy of, or modify, this frame)"
        n124 = call <vilib>:"Add State(s) to Queue__JKI_lib_State_Machine.vi"("State(s) in (\"\")"=w360) -> ("States Out"=w359:string)  [unwired: 14 in]
      }
      frame "Request: Handle Incoming" {
        n125 = Unbundle By Name(w362) -> ("project namespace"=w368:string, "Request.reply-to"=w364:string, "Client"=w370:refnum<class "Client.lvclass">, "Request.request"=w363:string)
        n126 = case shown="\"map\"" w363 {
          selector: w363 -> [w376 w381 w389]
          tunnel: w362 -> [_ w384 w391]
          tunnel: [w377 w382 w390] -> w361
          frame Default {
            w378 = "Unhandled Request"  # response
            n127 = Bundle(cluster=T4 {"request"="", "reply"=variant(string "")}, "request"=w376, "reply"=w378) -> (w377:T4)
          }
          frame "list-zones" {
            n128 = Unbundle By Name(w384) -> ("TrafficMap"=w385:refnum<class "TrafficMap.lvclass">)
            n129 = call "List Zones.vi"("TrafficMap in"=w385) -> ("Zones"=w383:string[])  [unwired: 7 in, 3 out]
            n130 = Bundle(cluster=T4 {"request"="", "reply"=variant(string "")}, "request"=w381, "reply"=w383) -> (w382:T4)
          }
          frame "map" {
            n131 = Unbundle By Name(w391) -> ("TrafficMap"=w387:refnum<class "TrafficMap.lvclass">)
            n132 = call "Read Map.vi"("TrafficMap in"=w387) -> ("Map"=w386:u16[][])  [unwired: 8 in, 2 out]
            n133 = Bundle(cluster=T4 {"request"="", "reply"=variant(string "")}, "request"=w389, "reply"=w386) -> (w390:T4)
          }
        }
        n134 = Format Into String(format string="%s/%s", w368, w364) -> (resulting string=w365:string)  [unwired: 2 in, 1 out]
        n135 = call <vilib>:"Publish.vi"("error in (no error)"=w367, "Payload"=w361, "Topic Name (empty: Payload name)"=w365, "Client in"=w370) -> ("error out"=w366:errorcluster, "Client out"=w371:refnum<class "Client.lvclass">)  [unwired: 5 in, 1 out]
        n136 = Bundle By Name(cluster=w362, "Client"=w371) -> (w373:T11)
        n137 = call <vilib>:"Add State(s) to Queue__JKI_lib_State_Machine.vi"("State(s) in (\"\")"=w375) -> ("States Out"=w374:string)  [unwired: 14 in]
      }
      frame "---------- MQTT ----------" {
        # "MQTT Separator\n(You can make a copy of, or modify, this frame)"
        n138 = call <vilib>:"Add State(s) to Queue__JKI_lib_State_Machine.vi"("State(s) in (\"\")"=w396) -> ("States Out"=w395:string)  [unwired: 14 in]
      }
      frame "MQTT: Create Client" {
        # "Set JKI-JSON as the Serializer Class"
        n139 = call <vilib>:"Create MQTT Client.vi"("error in (no error)"=w403) -> ("error out"=w398:errorcluster, "Client out"=w401:refnum<class "Client.lvclass">)  [unwired: 9 in]
        n140 = call <vilib>:"Set Serializer.vi"("error in (no error)"=w398, "Serializer (default: Flattened String)"=refnum<class "Serializer.JKI-JSON.lvclass"> refnum ("Serializer.JKI-JSON.lvclass"), "MQTT_Base"=w401) -> ("error out"=w397:errorcluster, "MQTT_Base out"=w400:refnum<class "Client.lvclass">)  [unwired: 7 in]
        n141 = Bundle By Name(cluster=w405, "Client"=w400) -> (w404:T11)
        n142 = call <vilib>:"Add State(s) to Queue__JKI_lib_State_Machine.vi"("State(s) in (\"\")"=w407) -> ("States Out"=w406:string)  [unwired: 14 in]
      }
      frame "MQTT: Register for Events" {
        n143 = Unbundle By Name(w416) -> ("Client"=w414:refnum<class "Client.lvclass">, "stop signal"=w408:refnum<user-event>)
        n144 = call <vilib>:"Read Public Events.vi"("error in (no error)"=w412, "Client in"=w414) -> ("error out"=w410:errorcluster, "Client Public Events"=w415:T13, "Client out"=w413:refnum<class "Client.lvclass">)  [unwired: 7 in]
        n145 = register-events(error in=w410, w415, w408) -> (reference out=w411:refnum<event-registration>, error out=w409:errorcluster)  [unwired: 1 in]
        n146 = Bundle By Name(cluster=w416, "Client"=w413) -> (w417:T11)
        n147 = call <vilib>:"Add State(s) to Queue__JKI_lib_State_Machine.vi"("State(s) in (\"\")"=w419) -> ("States Out"=w418:string)  [unwired: 14 in]
      }
      frame "MQTT: Connect" {
        n148 = Unbundle By Name(w440) -> ("server address"=w433:string, "Client"=w436:refnum<class "Client.lvclass">, "project namespace"=w425:string, "Client Name"=w424:string)
        n149 = call <vilib>:"Start.vi"("error in (no error)"=w435, "MQTT_Base in"=w436) -> ("error out"=w438:errorcluster, "MQTT_Base out"=w437:refnum<class "Client.lvclass">)  [unwired: 7 in, 1 out]
        n150 = call <vilib>:"Flatten To JSON String.vi"("Variant"=cluster{"message":string} {"message"="unexpected disconnection"}) -> ("JSON String"=w420:string)  [unwired: 9 in, 1 out]
        n151 = Format Into String(format string="%s/%s/will", w425, w424) -> (resulting string=w426:string)  [unwired: 2 in, 1 out]
        n152 = Bundle By Name(cluster=T5 {"Reserved"=FALSE, "Clean Session"=FALSE, "Will Flag"=FALSE, "Will QoS 1"=FALSE, "Will QoS 2"=FALSE, "Will Retain"=FALSE, "Password Flag"=FALSE, "User Name Flag"=FALSE} ("Connect Flags"), "Will Flag"=TRUE) -> (w428:T5)
        n153 = Bundle By Name(cluster=T6 {"Will Topic"="", "Will Message"="", "Username"="", "Password"=""} ("Payload"), "Will Topic"=w426, "Will Message"=w420) -> (w422:T6)
        n154 = call <vilib>:"Connect to Server.vi"("Connect Flags"=w428, "Keep Alive (s)"=u16 3600, "Payload"=w422, "error in (no error)"=w438, "address (localhost)"=w433, "Client in"=w437) -> ("error out"=w434:errorcluster, "Client out"=w432:refnum<class "Client.lvclass">)  [unwired: 2 in, 2 out]
        n155 = Bundle By Name(cluster=w440, "Client"=w432) -> (w441:T11)
        n156 = call <vilib>:"Add State(s) to Queue__JKI_lib_State_Machine.vi"("State(s) in (\"\")"=w443) -> ("States Out"=w442:string)  [unwired: 14 in]
      }
      frame "MQTT: Subscribe" {
        n157 = Unbundle By Name(w453) -> ("project namespace"=w450:string, "Client Name"=w449:string, "Client"=w448:refnum<class "Client.lvclass">)
        n158 = Format Into String(format string="%s/users/%s/#", w450, w449) -> (resulting string=w444:string)  [unwired: 2 in, 1 out]
        n159 = call <vilib>:"Subscribe (SingleTopic).vi"("error in (no error)"=w446, "Topic Filter"=w444, "MQTT_Base in"=w448) -> ("error out"=w445:errorcluster, "MQTT_Base out"=w447:refnum<class "Client.lvclass">)  [unwired: 7 in]
        n160 = Bundle By Name(cluster=w453, "Client"=w447) -> (w454:T11)
        n161 = call <vilib>:"Add State(s) to Queue__JKI_lib_State_Machine.vi"("State(s) in (\"\")"=w456) -> ("States Out"=w455:string)  [unwired: 14 in]
      }
      frame "MQTT: Unsubscribe" {
        n162 = Unbundle By Name(w466) -> ("project namespace"=w459:string, "Client Name"=w457:string, "Client"=w464:refnum<class "Client.lvclass">)
        n163 = Format Into String(format string="%s/users/%s/#", w459, w457) -> (resulting string=w458:string)  [unwired: 2 in, 1 out]
        n164 = call <vilib>:"Unsubscribe (SingleTopic).vi"("error in (no error)"=w462, "Topic Filter"=w458, "MQTT_Base in"=w464) -> ("error out"=w461:errorcluster, "MQTT_Base out"=w463:refnum<class "Client.lvclass">)  [unwired: 7 in]
        n165 = Bundle By Name(cluster=w466, "Client"=w463) -> (w467:T11)
        n166 = call <vilib>:"Add State(s) to Queue__JKI_lib_State_Machine.vi"("State(s) in (\"\")"=w469) -> ("States Out"=w468:string)  [unwired: 14 in]
      }
      frame "MQTT: Publish State" {
        n167 = Unbundle By Name(w481) -> ("project namespace"=w476:string, "Client Name"=w475:string, "Client"=w478:refnum<class "Client.lvclass">)
        n168 = Format Into String("car state") -> (resulting string=w470:string)  [unwired: 3 in, 1 out]
        n169 = Format Into String(format string="%s/users/%s/state", w476, w475) -> (resulting string=w474:string)  [unwired: 2 in, 1 out]
        n170 = call <vilib>:"Publish.vi"("error in (no error)"=w473, "Payload"=w470, "Topic Name (empty: Payload name)"=w474, "Client in"=w478) -> ("error out"=w472:errorcluster, "Client out"=w479:refnum<class "Client.lvclass">)  [unwired: 5 in, 1 out]
        n171 = Bundle By Name(cluster=w481, "Client"=w479) -> (w482:T11)
        n172 = call <vilib>:"Add State(s) to Queue__JKI_lib_State_Machine.vi"("State(s) in (\"\")"=w484) -> ("States Out"=w483:string)  [unwired: 14 in]
      }
      frame "MQTT: Publish Position" {
        n173 = Unbundle By Name(w496) -> ("project namespace"=w491:string, "Client Name"=w490:string, "Client"=w493:refnum<class "Client.lvclass">, "TrafficMap"=w486:refnum<class "TrafficMap.lvclass">)
        n174 = call "Read Position.vi"("TrafficMap in"=w486) -> ("Position"=w485:string)  [unwired: 8 in, 2 out]
        n175 = Format Into String(format string="%s/users/%s/position", w491, w490) -> (resulting string=w489:string)  [unwired: 2 in, 1 out]
        n176 = call <vilib>:"Publish.vi"("error in (no error)"=w488, "Payload"=w485, "Topic Name (empty: Payload name)"=w489, "Client in"=w493) -> ("error out"=w487:errorcluster, "Client out"=w494:refnum<class "Client.lvclass">)  [unwired: 5 in, 1 out]
        n177 = Bundle By Name(cluster=w496, "Client"=w494) -> (w497:T11)
        n178 = call <vilib>:"Add State(s) to Queue__JKI_lib_State_Machine.vi"("State(s) in (\"\")"=w499) -> ("States Out"=w498:string)  [unwired: 14 in]
      }
      frame "MQTT: RequestZoneList" {
        n179 = Unbundle By Name(w514) -> ("project namespace"=w502:string, "Client Name"=w501:string, "Client"=w511:refnum<class "Client.lvclass">)  [unwired: 1 out]
        n180 = Format Into String(format string="%s/users/%s/inbox", w502, w501) -> (resulting string=w504:string)  [unwired: 2 in, 1 out]
        n181 = Format Into String(format string="%s/traffic-data/request", w502) -> (resulting string=w509:string)  [unwired: 2 in, 1 out]
        n182 = Bundle By Name(cluster=T7 {"request"="", "reply-to"=""} ("Request Payload"), "request"="list-zones" ("Request"), "reply-to"=w504) -> (w506:T7)
        n183 = call <vilib>:"Publish.vi"("error in (no error)"=w508, "Payload"=w506, "Topic Name (empty: Payload name)"=w509, "Client in"=w511) -> ("error out"=w507:errorcluster, "Client out"=w512:refnum<class "Client.lvclass">)  [unwired: 5 in, 1 out]
        n184 = Bundle By Name(cluster=w514, "Client"=w512) -> (w515:T11)
        n185 = call <vilib>:"Add State(s) to Queue__JKI_lib_State_Machine.vi"("State(s) in (\"\")"=w517) -> ("States Out"=w516:string)  [unwired: 14 in]
      }
      frame "MQTT: RequestTrafficMap" {
        n186 = Unbundle By Name(w532) -> ("project namespace"=w520:string, "Client Name"=w519:string, "Client"=w529:refnum<class "Client.lvclass">)  [unwired: 1 out]
        n187 = Format Into String(format string="%s/users/%s/inbox", w520, w519) -> (resulting string=w522:string)  [unwired: 2 in, 1 out]
        n188 = Format Into String(format string="%s/traffic-data/request", w520) -> (resulting string=w527:string)  [unwired: 2 in, 1 out]
        n189 = Bundle By Name(cluster=T7 {"request"="", "reply-to"=""} ("Request Payload"), "request"="map" ("Request"), "reply-to"=w522) -> (w524:T7)
        n190 = call <vilib>:"Publish.vi"("error in (no error)"=w526, "Payload"=w524, "Topic Name (empty: Payload name)"=w527, "Client in"=w529) -> ("error out"=w525:errorcluster, "Client out"=w530:refnum<class "Client.lvclass">)  [unwired: 5 in, 1 out]
        n191 = Bundle By Name(cluster=w532, "Client"=w530) -> (w533:T11)
        n192 = call <vilib>:"Add State(s) to Queue__JKI_lib_State_Machine.vi"("State(s) in (\"\")"=w535) -> ("States Out"=w534:string)  [unwired: 14 in]
      }
      frame "MQTT: PublishConnectionMessage" {
        n193 = Unbundle By Name(w549) -> ("project namespace"=w544:string, "Client Name"=w543:string, "Client"=w546:refnum<class "Client.lvclass">, "Node type"=w539:T10)
        n194 = Format Into String(w539) -> (resulting string=w538:string)  [unwired: 3 in, 1 out]
        n195 = Format Into String(format string="%s/users/%s/connect", w544, w543) -> (resulting string=w542:string)  [unwired: 2 in, 1 out]
        n196 = Bundle(cluster=T8 {"Node type"=""} ("Connect payload"), "Node type"=w538) -> (w537:T8)
        n197 = call <vilib>:"Publish.vi"("error in (no error)"=w541, "Payload"=w537, "Topic Name (empty: Payload name)"=w542, "Client in"=w546) -> ("error out"=w540:errorcluster, "Client out"=w547:refnum<class "Client.lvclass">)  [unwired: 5 in, 1 out]
        n198 = Bundle By Name(cluster=w549, "Client"=w547) -> (w550:T11)
        n199 = call <vilib>:"Add State(s) to Queue__JKI_lib_State_Machine.vi"("State(s) in (\"\")"=w552) -> ("States Out"=w551:string)  [unwired: 14 in]
      }
      frame "MQTT: PublishDisconnectionMessage" {
        n200 = Unbundle By Name(w565) -> ("project namespace"=w560:string, "Client Name"=w559:string, "Client"=w562:refnum<class "Client.lvclass">)
        n201 = Format Into String(format string="%s/users/%s/disconnect", w560, w559) -> (resulting string=w558:string)  [unwired: 2 in, 1 out]
        n202 = call "Formatted Timestamp.vi"() -> ("String Formatted timestamp"=w554:string)  [unwired: 11 in]
        n203 = Bundle(cluster=T9 {"timestamp"=""} ("Disconnect payload"), "timestamp"=w554) -> (w553:T9)
        n204 = call <vilib>:"Publish.vi"("error in (no error)"=w557, "Payload"=w553, "Topic Name (empty: Payload name)"=w558, "Client in"=w562) -> ("error out"=w556:errorcluster, "Client out"=w563:refnum<class "Client.lvclass">)  [unwired: 5 in, 1 out]
        n205 = Bundle By Name(cluster=w565, "Client"=w563) -> (w566:T11)
        n206 = call <vilib>:"Add State(s) to Queue__JKI_lib_State_Machine.vi"("State(s) in (\"\")"=w568) -> ("States Out"=w567:string)  [unwired: 14 in]
      }
      frame "MQTT: Handle App Message" {
        n207 = Unbundle By Name(w575) -> ("Client Name"=w569:string, "Client"=w582:refnum<class "Client.lvclass">, "AppMessage"=w572:refnum<class "PUBLISH.lvclass">)
        n208 = call <vilib>:"Read Payload.vi"("ControlPacket in"=w572) -> ("Payload"=w571:u8[])  [unwired: 9 in, 1 out]
        n209 = call <vilib>:"getTopicName.vi"("PUBLISH in"=w572) -> ("Topic"=w581:string, "PUBLISH out"=w583:refnum<class "PUBLISH.lvclass">)  [unwired: 8 in, 1 out]
        "Topic" <- w581
        n210 = property on="Car Client Status" class="MCListbox (strict)"() -> ("ItemNames"=w579:string[][])  [unwired: 2 in, 2 out]
        n211 = Byte Array To String(unsigned byte array=w571) -> (string=→"Raw Packet String":string)
        n212 = call "topic_to_Array.vi"("Topic"=w581) -> ("Topic (Array)"=w585:string[])  [unwired: 10 in]
        n213 = Delete From Array(array=w585) -> (deleted portion=w584:string, array with subset deleted=w580:string[])  [unwired: 2 in]
        n214 = case shown="\"inbox\"" w584 {
          tunnel: w583 -> [w593 w598 w609 w647 w674 w699 w716]
          tunnel: w582 -> [w594 w599 w612 w646 w673 w698 _]
          tunnel: w580 -> [_ _ _ w645 w672 w697 w723]
          tunnel: w579 -> [w591 w602 w611 w635 w662 w689 w714]
          tunnel: [w591 w602 w611 w641 w668 w692 w718] -> w577
          tunnel: w575 -> [w590 w601 w604 w638 w665 w688 w713]
          tunnel: [w590 w600 w605 w638 w665 w688 w713] -> w574
          tunnel: [_ "Request: Handle Incoming" w603 _ _ _ _] -> w573
          tunnel: w569 -> [_ _ _ _ _ _ _]
          frame Default {
            n215 = call "Decode Publish Packet.vim"("PUBLISH"=w593, "Client in"=w594) -> ("Payload"=→"Payload":variant)  [unwired: 6 in, 3 out]
          }
          frame "request" {
            n216 = call "Decode Publish Packet.vim"("Payload type"=T7 {"request"="", "reply-to"=""} ("Request Payload"), "PUBLISH"=w598, "Client in"=w599) -> ("Payload"=w596:T7)  [unwired: 5 in, 3 out]
            n217 = Bundle By Name(cluster=w601, "Request"=w596) -> (w600:T11)
          }
          frame "inbox" {
            n218 = call "Decode Publish Packet.vim"("Payload type"=T4 {"request"="", "reply"=variant} ("Response Payload"), "PUBLISH"=w609, "Client in"=w612) -> ("Payload"=w608:T4)  [unwired: 5 in, 3 out]
            n219 = Unbundle(w608) -> ("request"=w607:string, "reply"=w606:variant)
            n220 = case shown="\"map\"" w607 {
              tunnel: w606 -> [_ w623 w633]
              tunnel: [w613 w617 w630] -> w605
              tunnel: w604 -> [w613 w615 w628]
              tunnel: [_ "UI: Update Zone List" "UI: Update Zone Map"] -> w603
              frame "False", Default {
              }
              frame "list-zones" {
                w620 = string[] []
                n221 = Unbundle By Name(w615) -> ("TrafficMap"=w614:refnum<class "TrafficMap.lvclass">)
                n222 = call <vilib>:"Adapt To Type.vi"("Type and Defaults"=w620, "Variant in"=w623) -> ("error out"=w622:errorcluster, "Variant out"=w621:variant)  [unwired: 8 in]
                n223 = Variant To Data(error in=w622, type=w620, Variant=w621) -> (data=w618:string[])  [unwired: 1 out]
                n224 = call "Create TrafficMap.vi"("TrafficMap in"=w614, "Zones"=w618) -> ("TrafficMap"=w619:refnum<class "TrafficMap.lvclass">)  [unwired: 8 in, 1 out]
                n225 = Bundle By Name(cluster=w615, "TrafficMap"=w619) -> (w617:T11)
              }
              frame "map" {
                w627 = u16[][] []  # Map
                n226 = Unbundle By Name(w628) -> ("TrafficMap"=w626:refnum<class "TrafficMap.lvclass">)
                n227 = call <vilib>:"Adapt To Type.vi"("Type and Defaults"=w627, "Variant in"=w633) -> ("error out"=w632:errorcluster, "Variant out"=w631:variant)  [unwired: 8 in]
                n228 = Variant To Data(error in=w632, type=w627, Variant=w631) -> (data=w625:u16[][])  [unwired: 1 out]
                n229 = call "Write Map.vi"("Map"=w625, "TrafficMap in"=w626) -> ("TrafficMap out"=w624:refnum<class "TrafficMap.lvclass">)  [unwired: 8 in, 1 out]
                n230 = Bundle By Name(cluster=w628, "TrafficMap"=w624) -> (w630:T11)
              }
            }
          }
          frame "state" {
            n231 = Delete From Array(array=w645) -> (deleted portion=w642:string)  [unwired: 2 in, 1 out]
            n232 = Index Array(array=w635, index (col)=0 ("disabled index (col)")) -> (element=w643:string[])  [unwired: 1 in]
            n233 = call "Decode Publish Packet.vim"("Payload type"="", "PUBLISH"=w647, "Client in"=w646) -> ("Payload"=w639:string)  [unwired: 5 in, 3 out]
            n234 = Search 1D Array(1D array=w643, element=w642) -> (index of element=w637:i32)  [unwired: 1 in]
            n235 = Index Array(array=w635, index (row)=w637, index (col)=2) -> (element=w634:string)
            n236 = case shown="-1" w637 {
              selector: w637 -> [_ w655]
              tunnel: [w652 w657] -> w641
              tunnel: w635 -> [w651 w658]
              tunnel: w639 -> [w650 w660]
              tunnel: w642 -> [w649 w659]
              tunnel: w634 -> [w648 w654]
              frame -1 {
                n237 = Build Array(w649, w650, w648) -> (w653:string[])
                n238 = Build Array (concatenate)(w653, w651) -> (w652:string[][])
              }
              frame Default {
                n239 = Build Array(w659, w660, w654) -> (w656:string[])
                n240 = Replace Array Subset(array=w658, new element=w656, index (row)=w655) -> (w657:string[][])  [unwired: 1 in]
              }
            }
          }
          frame "position" {
            n241 = Delete From Array(array=w672) -> (deleted portion=w669:string)  [unwired: 2 in, 1 out]
            n242 = Index Array(array=w662, index (col)=0 ("disabled index (col)")) -> (element=w670:string[])  [unwired: 1 in]
            n243 = call "Decode Publish Packet.vim"("Payload type"="", "PUBLISH"=w674, "Client in"=w673) -> ("Payload"=w666:string)  [unwired: 5 in, 3 out]
            n244 = Search 1D Array(1D array=w670, element=w669) -> (index of element=w664:i32)  [unwired: 1 in]
            n245 = Index Array(array=w662, index (row)=w664, index (col)=1) -> (element=w661:string)
            n246 = case shown="Default" w664 {
              selector: w664 -> [_ w683]
              tunnel: [w679 w685] -> w668
              tunnel: w662 -> [w678 w686]
              tunnel: w666 -> [w676 w681]
              tunnel: w669 -> [w677 w687]
              tunnel: w661 -> [w675 w682]
              frame -1 {
                n247 = Build Array(w677, w675, w676) -> (w680:string[])
                n248 = Build Array (concatenate)(w680, w678) -> (w679:string[][])
              }
              frame Default {
                n249 = Build Array(w687, w682, w681) -> (w684:string[])
                n250 = Replace Array Subset(array=w686, new element=w684, index (row)=w683) -> (w685:string[][])  [unwired: 1 in]
              }
            }
          }
          frame "disconnect" {
            n251 = Delete From Array(array=w697) -> (deleted portion=w694:string)  [unwired: 2 in, 1 out]
            n252 = Index Array(array=w689, index (col)=0 ("disabled index (col)")) -> (element=w695:string[])  [unwired: 1 in]
            n253 = call "Decode Publish Packet.vim"("Payload type"="", "PUBLISH"=w699, "Client in"=w698) -> ("Payload"=w690:string)  [unwired: 5 in, 3 out]
            n254 = Search 1D Array(1D array=w695, element=w694) -> (index of element=w693:i32)  [unwired: 1 in]
            n255 = case shown="Default" w693 {
              selector: w693 -> [_ w710]
              tunnel: [w704 w712] -> w692
              tunnel: w689 -> [w703 w711]
              tunnel: w690 -> [w700 w706]
              tunnel: w694 -> [w702 _]
              frame -1 {
                n256 = Build Array(w702, "" ("element"), w700) -> (w705:string[])
                n257 = Build Array (concatenate)(w705, w703) -> (w704:string[][])
              }
              frame Default {
                n258 = Index Array(array=w711, index (row)=w710) -> (element=w709:string[])  [unwired: 1 in]
                n259 = Replace Array Subset(array=w709, new element=w706, index=2) -> (w707:string[])
                n260 = Replace Array Subset(array=w711, new element=w707, index (row)=w710) -> (w712:string[][])  [unwired: 1 in]
              }
            }
          }
          frame "will" {
            n261 = Delete From Array(array=w723) -> (deleted portion=w720:string)  [unwired: 2 in, 1 out]
            n262 = Index Array(array=w714, index (col)=0 ("disabled index (col)")) -> (element=w721:string[])  [unwired: 1 in]
            n263 = call <vilib>:"Read Payload.vi"("ControlPacket in"=w716) -> ("Payload"=w717:u8[])  [unwired: 9 in, 1 out]
            n264 = Search 1D Array(1D array=w721, element=w720) -> (index of element=w719:i32)  [unwired: 1 in]
            n265 = Byte Array To String(unsigned byte array=w717) -> (string=w715:string)
            n266 = case shown="Default" w719 {
              selector: w719 -> [_ w732]
              tunnel: [w728 w734] -> w718
              tunnel: w714 -> [w727 w735]
              tunnel: w715 -> [w724 w731]
              tunnel: w720 -> [w726 w736]
              frame -1 {
                n267 = Build Array(w726, "" ("element"), w724) -> (w729:string[])
                n268 = Build Array (concatenate)(w729, w727) -> (w728:string[][])
              }
              frame Default {
                n269 = Build Array(w736, "" ("element"), w731) -> (w733:string[])
                n270 = Replace Array Subset(array=w735, new element=w733, index (row)=w732) -> (w734:string[][])  [unwired: 1 in]
              }
            }
          }
        }
        n271 = Array Subset(array=w577, length (row)=50 ("length")) -> (w576:string[][])  [unwired: 3 in]
        n272 = property on="Car Client Status" class="MCListbox (strict)"("ItemNames"=w576) -> ()  [unwired: 2 in, 2 out]
        n273 = call <vilib>:"Add State(s) to Queue__JKI_lib_State_Machine.vi"("State(s) in Front (\"\")"=w573, "State(s) in (\"\")"=w589) -> ("States Out"=w588:string)  [unwired: 13 in]
      }
      frame "MQTT: Disconnect" {
        n274 = Unbundle By Name(w744) -> ("Client"=w742:refnum<class "Client.lvclass">)
        n275 = call <vilib>:"Disconnect from Server.vi"("error in (no error)"=w737, "Client in"=w742) -> ("error out"=w738:errorcluster, "Client out"=w741:refnum<class "Client.lvclass">)  [unwired: 7 in, 1 out]
        n276 = call <vilib>:"Stop.vi"("error in (no error)"=w738, "MQTT_Base in"=w741) -> ("error out"=w739:errorcluster, "MQTT_Base out"=w740:refnum<class "Client.lvclass">)  [unwired: 7 in, 1 out]
        n277 = Bundle By Name(cluster=w744, "Client"=w740) -> (w745:T11)
        n278 = call <vilib>:"Add State(s) to Queue__JKI_lib_State_Machine.vi"("State(s) in (\"\")"=w747) -> ("States Out"=w746:string)  [unwired: 14 in]
      }
      frame "MQTT: Unregister" {
        n279 = Unregister For Events(event registration refnum=w751, error in=w750) -> (error out=w749:errorcluster)
        n280 = call <vilib>:"Add State(s) to Queue__JKI_lib_State_Machine.vi"("State(s) in (\"\")"=w753) -> ("States Out"=w752:string)  [unwired: 14 in]
      }
      frame "MQTT: Destroy Client" {
        n281 = Unbundle By Name(w758) -> ("Client"=w757:refnum<class "Client.lvclass">)
        n282 = call-dynamic "Destroy.vi"("error in (no error)"=w756, "MQTT_Base in"=w757) -> ("error out"=w755:errorcluster)  [unwired: 8 in, 1 out]
        n283 = call <vilib>:"Add State(s) to Queue__JKI_lib_State_Machine.vi"("State(s) in (\"\")"=w760) -> ("States Out"=w759:string)  [unwired: 14 in]
      }
    }
  }
